vi "Initialize.vi"(8 "error in (no error)":errorcluster, 9 "transceiver settings":T1, 10 "Transfer Groups Configurations":refnum<class "Transfer Group Configuration.lvclass">[](array[class]), 11 "UDP in":refnum<class "UDP Transceiver.lvclass">) -> (0 "error out":errorcluster, 3 "UDP out":refnum<class "UDP Transceiver.lvclass">)   [LabVIEW 2017, in "UDP Transceiver.lvlib" / "UDP Transceiver.lvclass"]
uses:
  UDP Transceiver.lvclass
  Builds/Data Sharing Framework/Current/Data Sharing Framework Core/DSF Core.lvlibp/Shared/Classes/Transfer Group/Transfer Group Configuration.lvclass
  Builds/Data Sharing Framework/Current/Data Sharing Framework Core/DSF Core.lvlibp/DSF Configuration API/Public/Controls/DSF Settings Info.ctl
  UDP Transceiver.lvclass/UDP Transceiver.ctl
  Builds/Data Sharing Framework/Current/Data Sharing Framework Core/DSF Core.lvlibp
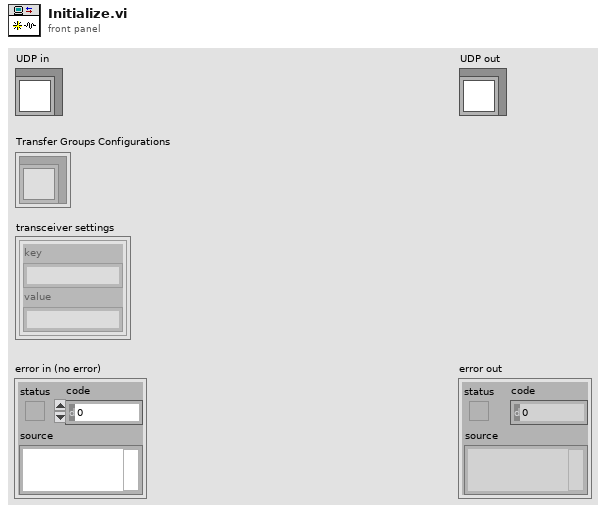
[diagram p1: front panel]
types:
  T1 = typedef "DSF Core.lvlibp/DSF Settings Info.ctl" = cluster{"key":string, "value":string}[]
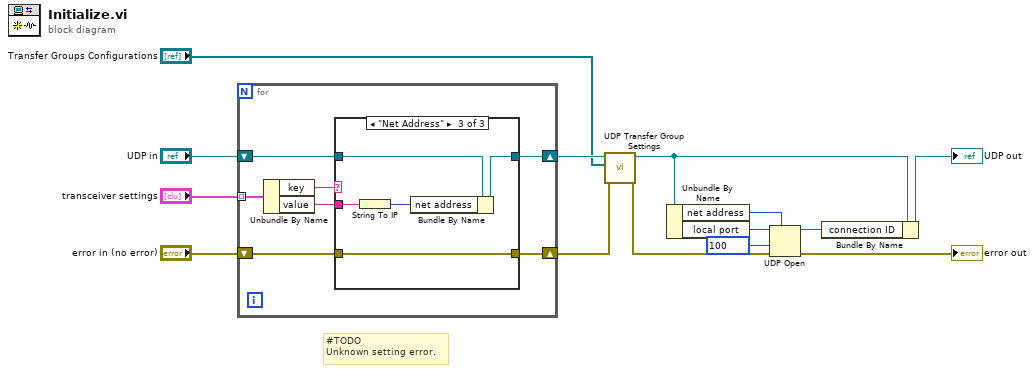
[diagram p0: block diagram]
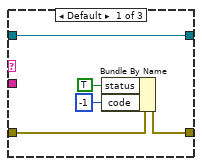
[diagram p2: hidden frame]
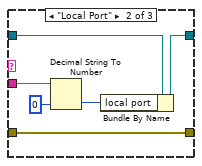
[diagram p3: hidden frame]
diagram:
  # "#TODO\nUnknown setting error."
  n1 = for {
    tunnel: "transceiver settings" -> [w21] mode=indexing
    shift-right: [w17] -> w14
    shift-left: "UDP in" -> [w18]
    shift-right: [w15] -> w13
    shift-left: "error in (no error)" -> [w16]
    n2 = Unbundle By Name(w21) -> ("key"=w20:string, "value"=w19:string)
    n3 = case shown="\"Net Address\"" w20 {
      tunnel: w19 -> [_ w31 w34]
      tunnel: w18 -> [w26 w30 w37]
      tunnel: [w26 w29 w36] -> w17
      tunnel: w16 -> [w25 w28 w35]
      tunnel: [w24 w28 w35] -> w15
      frame Default {
        n4 = Bundle By Name(cluster=w25, "status"=TRUE, "code"=-1) -> (w24:errorcluster)
      }
      frame "Local Port" {
        n5 = Decimal String To Number(string=w31, default (0L)=u16 0 ("default (0 I32)")) -> (number=w27:u16)  [unwired: 1 in, 1 out]
        n6 = Bundle By Name(cluster=w30, "local port"=w27) -> (w29:refnum<class "UDP Transceiver.lvclass">)
      }
      frame "Net Address" {
        n7 = String To IP(1:w34) -> (0:w33:u32)
        n8 = Bundle By Name(cluster=w37, "net address"=w33) -> (w36:refnum<class "UDP Transceiver.lvclass">)
      }
    }
  }
  n9 = call "UDP Transfer Group Settings.vi"("error in (no error)"=w13, "Transfer Groups Configurations"="Transfer Groups Configurations", "UDP Transceiver in"=w14) -> ("error out"=w12:errorcluster, "UDP Transceiver out"=w11:refnum<class "UDP Transceiver.lvclass">)  [unwired: 7 in]
  n10 = Unbundle By Name(w11) -> ("net address"=w7:u32, "local port"=w10:u16)
  n11 = UDP Open(7:w7, 8:w12, 9:100 ("timeout ms (25000)"), 11:w10) -> (port=w8:refnum<k16>, 0:→"error out":errorcluster)  [unwired: 1 in, 1 out]
  n12 = Bundle By Name(cluster=w11, "connection ID"=w8) -> (→"UDP out":refnum<class "UDP Transceiver.lvclass">)
